vi "CAN_reset.vi"(8 "error in":errorcluster, 9 "Reset":bool, 10 "Node ID":u8=3, 11 "CAN Session In":refnum<class "sbCANopenBaseClass.lvclass">) -> (0 "error out":errorcluster, 3 "CANopen Session Out":refnum<class "sbCANopenBaseClass.lvclass">)   [LabVIEW 2017]
doc: "Initializes an EPOS2 drive and returns a node specific CANopen session reference."
uses:
  <vilib>/addons/Maxon Motor/EPOS2 CANopen/CANopen/sbCANopenBaseClass.lvclass
  <vilib>/addons/Maxon Motor/EPOS2 CANopen/EPOS2 Support Files/Typedefs/EPOS2 Control Word IPM.ctl
  <vilib>/addons/Maxon Motor/EPOS2 CANopen/CANopen/TypeDefs/sdCANopenNMTCommand.ctl
  <vilib>/addons/Maxon Motor/EPOS2 CANopen/EPOS2 Support Files/SubVIs/EPOS2 Read Status Word IPM.vi
  <vilib>/addons/Maxon Motor/EPOS2 CANopen/EPOS2 Support Files/SubVIs/EPOS2 Write Control Word IPM.vi
  <vilib>/addons/Maxon Motor/EPOS2 CANopen/EPOS2 Library.lvlib
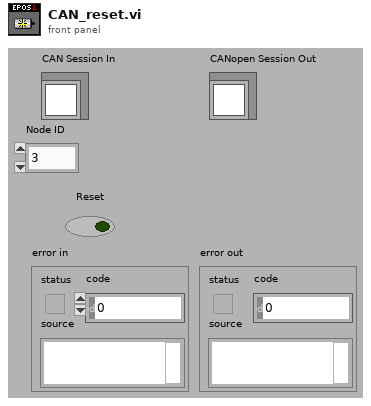
[diagram p1: front panel]
types:
  T1 = typedef "sdCANopenNMTCommand.ctl" = enum16{"Start", "Stop", "Enter Pre-Operational State", "Reset", "Reset Communication"}
  T2 = typedef "EPOS2 Library.lvlib/EPOS2 Control Word IPM.ctl" = cluster{"Switch On":bool, "Enable Voltage":bool, "Quick Stop":bool, "Enable Operation":bool, "Enable IPM":bool, "Reserved 1":bool, "Reserved 2":bool, "Fault Reset":bool, "Halt":bool}
  T3 = typedef "EPOS2 Library.lvlib/EPOS2 Status Word IPM.ctl" = cluster{"Ready to Switch On":bool, "Switched On":bool, "Operation Enable":bool, "Fault":bool, "Voltage Enabled":bool, "Quick Stop":bool, "Switch On Disable":bool, "Warning":bool, "Offset Current Measured":bool, "Remote":bool, "Target Reached":bool, "Internal Limit Active":bool, "IPM Active":bool, "Reserved":bool, "Refresh Cycle of Power Stage":bool, "Position Reference to Home Position":bool}
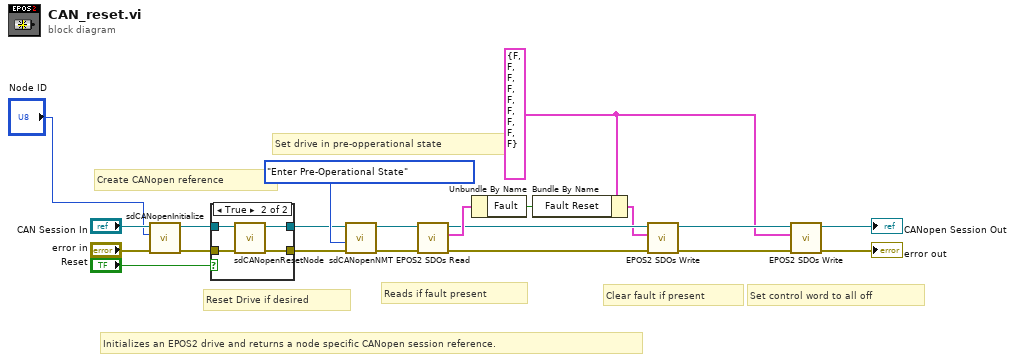
[diagram p0: block diagram]
diagram:
  w5 = T2 {"Switch On"=FALSE, "Enable Voltage"=FALSE, "Quick Stop"=FALSE, "Enable Operation"=FALSE, "Enable IPM"=FALSE, "Reserved 1"=FALSE, "Reserved 2"=FALSE, "Fault Reset"=FALSE, "Halt"=FALSE} ("IPM Control Word")
  # "Initializes an EPOS2 drive and returns a node specific CANopen session reference."
  # "Create CANopen reference"
  # "Reset Drive if desired"
  # "Clear fault if present"
  # "Reads if fault present"
  # "Set control word to all off"
  # "Set drive in pre-opperational state"
  n1 = call-dynamic "sdCANopenInitialize.vi"("error in (no error)"="error in", "Node ID"="Node ID", "sbCANopenBaseClass in"="CAN Session In") -> ("error out"=w10:errorcluster, "sbCANopenBaseClass out"=w8:refnum<class "sbCANopenBaseClass.lvclass">)  [unwired: 7 in]
  n2 = case shown="True" "Reset" {
    tunnel: w10 -> [w22 w27]
    tunnel: [w22 w26] -> w9
    tunnel: w8 -> [w23 w25]
    tunnel: [w23 w24] -> w3
    frame False {
    }
    frame True {
      n3 = call <vilib>:"sdCANopenResetNode.vi"("error in"=w27, "CANopen Session In"=w25) -> ("error out"=w26:errorcluster, "CANopen Session Out"=w24:refnum<class "sbCANopenBaseClass.lvclass">)  [unwired: 8 in]
    }
  }
  n4 = call-dynamic "sdCANopenNMT.vi"("error in (no error)"=w9, "NMT Command"=sdCANopenNMTCommand."Enter Pre-Operational State", "sbCANopenBaseClass in"=w3) -> ("error out"=w20:errorcluster, "sbCANopenBaseClass out"=w2:refnum<class "sbCANopenBaseClass.lvclass">)  [unwired: 7 in]
  n5 = call-poly <vilib>:"EPOS2 SDOs Read.vi"("error in"=w20, "CANopen Session In"=w2) -> ("error out"=w13:errorcluster, "Status Word IPM"=w19:T3, "CANopen Session Out"=w12:refnum<class "sbCANopenBaseClass.lvclass">)  [unwired: 7 in]
  n6 = Unbundle By Name(w19) -> ("Fault"=w14:bool)
  n7 = Bundle By Name(cluster=w5, "Fault Reset"=w14) -> (w6:T2)
  n8 = call-poly <vilib>:"EPOS2 SDOs Write.vi"("error in"=w13, "IPM Control Word"=w6, "CANopen Session In"=w12) -> ("error out"=w17:errorcluster, "CANopen Session Out"=w18:refnum<class "sbCANopenBaseClass.lvclass">)  [unwired: 7 in]
  n9 = call-poly <vilib>:"EPOS2 SDOs Write.vi"("error in"=w17, "IPM Control Word"=w5, "CANopen Session In"=w18) -> ("error out"=→"error out":errorcluster, "CANopen Session Out"=→"CANopen Session Out":refnum<class "sbCANopenBaseClass.lvclass">)  [unwired: 7 in]
